vi "Read InitVal.vi"(8 "error in (no error)":errorcluster, 11 "O3 Generator Power STEP in":refnum<class "O3 Generator Power STEP.lvclass">) -> (0 "error out":errorcluster, 2 "InitVal":u8, 3 "O3 Generator Power STEP out":refnum<class "O3 Generator Power STEP.lvclass">)   [LabVIEW 2014, in "O3 Generator Power STEP.lvclass"]
uses:
  O3 Generator Power STEP.lvclass
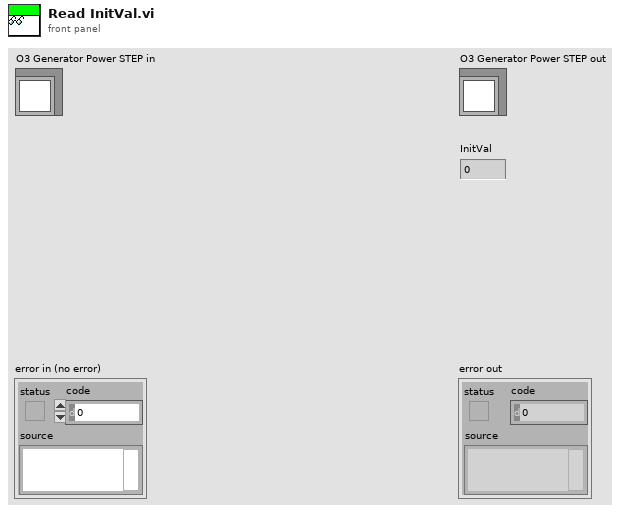
[diagram p1: front panel]
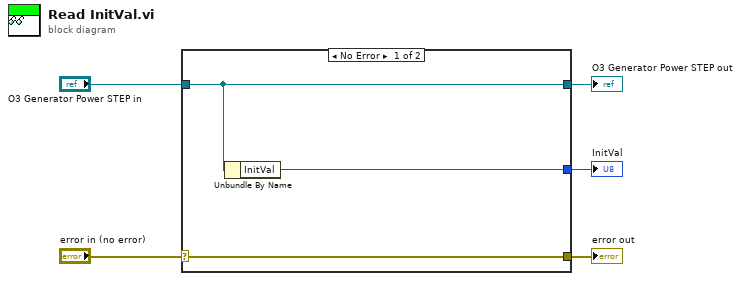
[diagram p0: block diagram]
diagram:
  n1 = case shown="No Error" "error in (no error)" {
    selector: "error in (no error)" -> [w8 w9]
    tunnel: [w8 w9] -> w4
    tunnel: [w7 w10] -> w2
    tunnel: "O3 Generator Power STEP in" -> [w7 w10]
    tunnel: [w6 _] -> w1
    frame No Error {
      n2 = Unbundle By Name(w7) -> ("InitVal"=w6:u8)
    }
    frame Error {
    }
  }
  "error out" <- w4
  "O3 Generator Power STEP out" <- w2
  "InitVal" <- w1
